vi "Read SampleClock.vi"(8 "error in (no error)":errorcluster, 11 "NiDaqMx in":refnum<class "NiDaqMx.lvclass">) -> (0 "error out":errorcluster, 2 "SampleClock":T1 {"sample mode" items=["Finite Samples"=10178, "Continuous Samples"=10123, "Hardware Timed Single Point"=12522]; "TimebaseRate" format="%#_6p"}, 3 "NiDaqMx out":refnum<class "NiDaqMx.lvclass">)   [LabVIEW 2018, in "DigitizerPlugins.lvlib" / "NiDaqMx.lvclass"]
uses:
  NiDaqMx.lvclass
  SampleClock.ctl
  NiDaqMx.lvclass/NiDaqMx.ctl
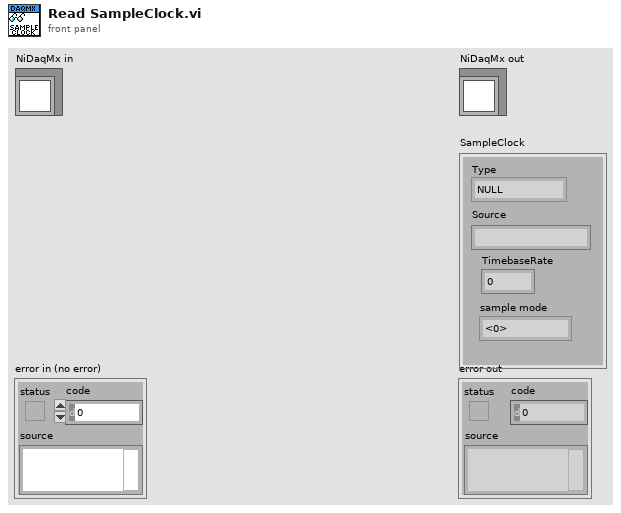
[diagram p1: front panel]
types:
  T1 = typedef "DigitizerPlugins.lvlib/NiDaqMx.lvclass/SampleClock.ctl" = cluster{"Type":enum16{"NULL", "Onboard", "External", "Software", "Interval"}, "Source":string, "TimebaseRate":dbl, "sample mode":i32}
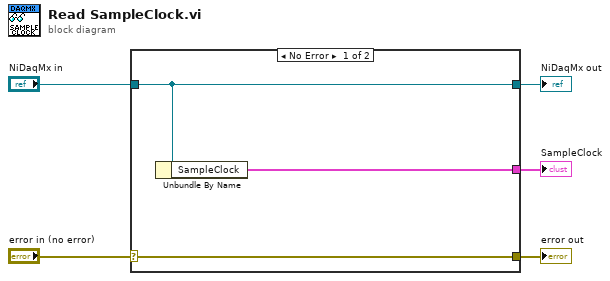
[diagram p0: block diagram]
diagram:
  n1 = case shown="No Error" "error in (no error)" {
    selector: "error in (no error)" -> [w8 w9]
    tunnel: [w8 w9] -> w4
    tunnel: [w7 w10] -> w2
    tunnel: "NiDaqMx in" -> [w7 w10]
    tunnel: [w6 _] -> w1
    frame No Error {
      n2 = Unbundle By Name(w7) -> ("SampleClock"=w6:T1)
    }
    frame Error {
    }
  }
  "error out" <- w4
  "NiDaqMx out" <- w2
  "SampleClock" <- w1
